vi "Configure Current Limit.vi"(8 "error in (no error)":errorcluster, 9 "Current Limit (0.00 A)":dbl format="%.2g", 11 "VISA resource name":refnum<visa-resource-name>) -> (0 "error out":errorcluster, 1 "chaîne concaténée":string, 3 "VISA resource name out":refnum<visa-resource-name>)   [LabVIEW 2020]
doc: "Configures the current limit. Specify the output current limit value and the behavior of the power supply when the output current is greater than or equal to that value."
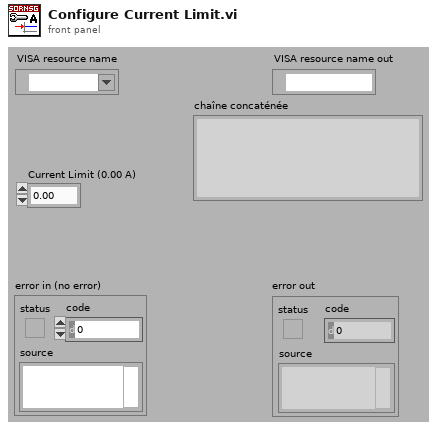
[diagram p1: front panel]
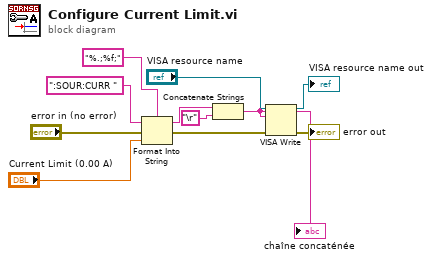
[diagram p0: block diagram]
diagram:
  n1 = Format Into String(format string="%.;%f;", initial string=":SOUR:CURR ", error in="error in (no error)", "Current Limit (0.00 A)") -> (resulting string=w4:string, error out=w5:errorcluster)
  n2 = Concatenate Strings(w4, "\r") -> (w2:string)
  "chaîne concaténée" <- w2
  n3 = VISA Write(VISA resource name="VISA resource name", write buffer=w2, error in (no error)=w5) -> (VISA resource name out=→"VISA resource name out":refnum<visa-resource-name>, error out=→"error out":errorcluster)  [unwired: 1 out]
